vi "Restart System.vi"(8 "error in":errorcluster, 11 "tCRD in":refnum<class "Aircraft OPCCRD.lvclass">) -> (0 "error out":errorcluster, 3 "tCRD out":refnum<class "Aircraft OPCCRD.lvclass">)   [LabVIEW 2015, in "Aircraft OPCCRD.lvclass"]
doc: "If a restart has been requested, then we will grab a single record and check that record for a discontinuity. If one exists, retrieve the number of elements from the CRD Data buffer up to the location of the discontinuity. Reset the Restart Requested? flag."
uses:
  Aircraft OPCCRD.lvclass
  Reusable/Instrument/Instrument.lvclass/Instrument.ctl
  Aircraft OPCCRD.lvclass/Aircraft OPCCRD.ctl
  Reusable/Instrument/Write Restart Requested_.vi
  Reusable/Instrument/Read Restart Requested_.vi
  Accessors/Read FPGA Ref.vi
  Accessors/Read SamplesPerRep.vi
  Reusable/Instrument/Read Log Session.vi
  <vilib>/Utility/error.llb/Error Cluster From Error Code.vi
  <vilib>/rvi/errors/niLvFpgaAdjustHostInterfaceError.vi
  tFPGA Ref.ctl
  <userlib>/_Session Fwk/Session - Root.lvclass
  <vilib>/rvi/interface/nirviMethod/nirviMethod.xnode
  FPGA Bitfiles/Aircraft OPCRD Server.lvbitx
  <vilib>/FPGAPlugInAG/sbRIO-9636/niLvFpga_ReadFifo_sbRIO-9636.vi
  <vilib>/rvi/errors/niLvFpgaMergeErrorWithErrorCode.vi
  Reusable/Session Log/System Log.lvclass
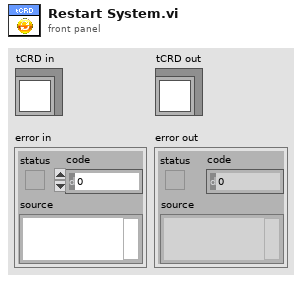
[diagram p1: front panel]
types:
  T1 = typedef "Aircraft OPCCRD.lvclass/tFPGA Ref.ctl" = refnum<k20>
  T2 = typedef "Session - Root.lvclass/Session Handle.ctl" = refnum<data-value>
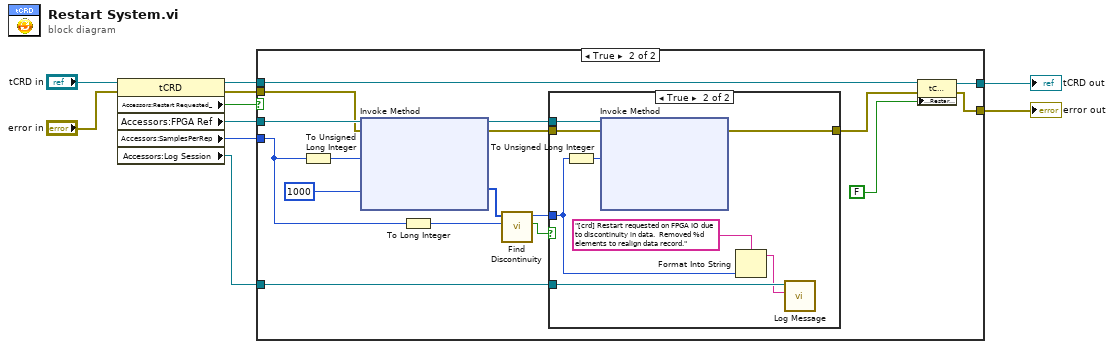
[diagram p0: block diagram]
diagram:
  n1 = property class="tCRD"(reference="tCRD in", error in="error in") -> (reference out=w3:refnum<class "Aircraft OPCCRD.lvclass">, error out=w5:errorcluster, "Accessors:Restart Requested_"=w8:bool, "Accessors:FPGA Ref"=w7:T1, "Accessors:SamplesPerRep"=w6:u16, "Accessors:Log Session"=w1:T2)
  n2 = case shown="True" w8 {
    tunnel: w7 -> [_ w29]
    tunnel: w6 -> [_ w15]
    tunnel: w5 -> [w12 w22]
    tunnel: [w12 w17] -> w4
    tunnel: w3 -> [w11 w21]
    tunnel: [w11 w19] -> w2
    tunnel: w1 -> [_ w13]
    frame False {
    }
    frame True {
      n3 = To Unsigned Long Integer(number=w15) -> (unsigned 32bit integer=w16:u32)
      n4 = xnode "Invoke Method"("FPGA VI Reference In"=w29, "error in"=w22, "Number of Elements"=w16, "Timeout (ms)"=1000) -> ("FPGA VI Reference Out"=w26:T1, "error out"=w23:errorcluster, "Data"=w27:i16[])  [unwired: 1 out]
      n5 = To Long Integer(number=w15) -> (32bit integer=w14:i32)
      n6 = call "Find Discontinuity.vi"("Single Record"=w14, "Data"=w27) -> ("Discontinuity Detected"=w25:bool, "cIndex"=w24:i32)  [unwired: 8 in]
      n7 = case shown="True" w25 {
        tunnel: w26 -> [_ w38]
        tunnel: w24 -> [_ w32]
        tunnel: w23 -> [w30 w37]
        tunnel: [w30 w36] -> w18
        tunnel: w13 -> [_ w34]
        frame False {
        }
        frame True {
          n8 = To Unsigned Long Integer(number=w32) -> (unsigned 32bit integer=w35:u32)
          n9 = xnode "Invoke Method"("FPGA VI Reference In"=w38, "error in"=w37, "Number of Elements"=w35) -> ("error out"=w36:errorcluster)  [unwired: 1 in, 3 out]
          n10 = Format Into String(format string="[crd] Restart requested on FPGA IO due to discontinuity in data.  Removed %d elements to realign data record." ("MSG In"), w32) -> (resulting string=w31:string)  [unwired: 2 in, 1 out]
          n11 = call "Log Message.vi"("MSG In"=w31, "session in"=w34) -> ()  [unwired: 8 in, 2 out]
        }
      }
      n12 = property class="tCRD"(reference=w21, error in=w18, "Accessors:Restart Requested_"=FALSE ("Restart Requested_")) -> (reference out=w19:refnum<class "Aircraft OPCCRD.lvclass">, error out=w17:errorcluster)
    }
  }
  "error out" <- w4
  "tCRD out" <- w2
